vi "get_waveform.vi"(0 "NInstrSim_ReadStatus":refnum<class "NInstrSim_ReadStatus.lvclass">, 5 "error in (no error)":errorcluster) -> (14 "dup NInstrSim_ReadStatus":refnum<class "NInstrSim_ReadStatus.lvclass">, 16 "Waveform":waveform(dbl), 19 "error out":errorcluster)   [LabVIEW 2009, in "HB_Device_Examples.lvlib" / "NInstrSim_ReadStatus.lvclass"]
doc: "This VI retruns the result of the Waveform Measurement."
uses:
  NInstrSim_ReadStatus.lvclass
  NInstrSim_ReadStatus.lvclass/NInstrSim_ReadStatus.ctl
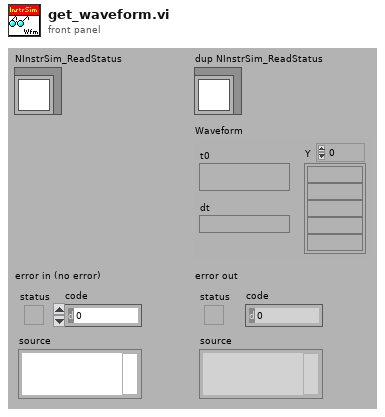
[diagram p1: front panel]
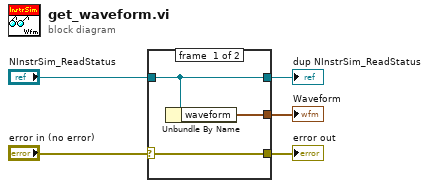
[diagram p0: block diagram]
diagram:
  n1 = case shown="No Error" "error in (no error)" {
    selector: "error in (no error)" -> [w8 w9]
    tunnel: [w8 w9] -> w4
    tunnel: [w7 w10] -> w2
    tunnel: "NInstrSim_ReadStatus" -> [w7 w10]
    tunnel: [w6 _] -> w1
    frame #0 {
      n2 = Unbundle By Name(w7) -> ("waveform"=w6:waveform(dbl))
    }
    frame #1 {
    }
  }
  "error out" <- w4
  "dup NInstrSim_ReadStatus" <- w2
  "Waveform" <- w1
